vi "Warning Leve Judge.vi"(9 "Limit":T1, 10 "key not found?":bool, 11 "Data":string) -> (2 "level":enum16{"", "Ⅰ", "Ⅱ", "Ⅲ", "Ⅳ", "Ⅴ"}(ring), 3 "字符串":string)   [LabVIEW 2020]
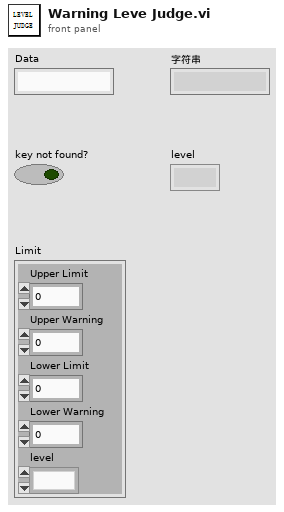
[diagram p1: front panel]
types:
  T1 = cluster{"Upper Limit":dbl, "Upper Warning":dbl, "Lower Limit":dbl, "Lower Warning":dbl, "level":enum16{"", "Ⅰ", "Ⅱ", "Ⅲ", "Ⅳ", "Ⅴ"}}
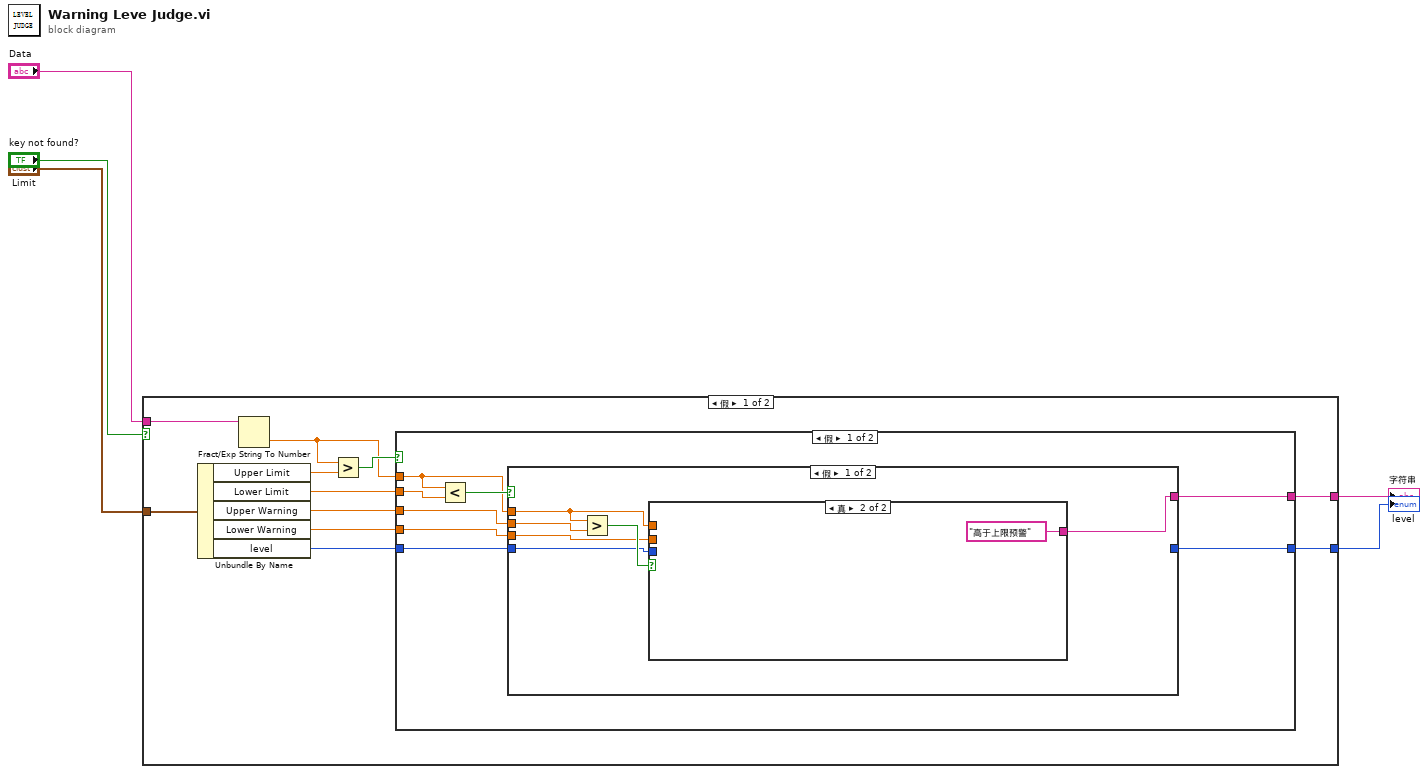
[diagram p0: block diagram]
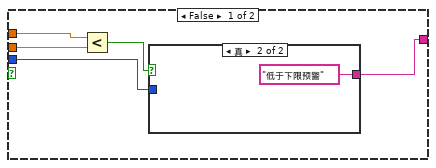
[diagram p2: hidden frame]
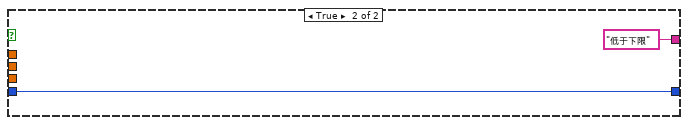
[diagram p4: hidden frame]
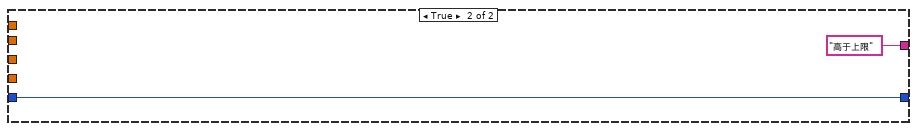
[diagram p5: hidden frame]
diagram:
  n1 = case shown="假" "key not found?" {
    tunnel: "Limit" -> [w16 _]
    tunnel: "Data" -> [w15 _]
    tunnel: [w12 _] -> w3
    tunnel: [w6 _] -> w4
    frame False {
      n2 = Unbundle By Name(w16) -> ("Upper Limit"=w14:dbl, "Lower Limit"=w10:dbl, "Upper Warning"=w9:dbl, "Lower Warning"=w8:dbl, "level"=w7:enum16{"", "Ⅰ", "Ⅱ", "Ⅲ", "Ⅳ", "Ⅴ"})
      n3 = Fract/Exp String To Number(string=w15) -> (number=w11:dbl)  [unwired: 3 in, 1 out]
      n4 = Greater?(x=w11, y=w14) -> (0:w13:bool)
      n5 = case shown="假" w13 {
        tunnel: [w22 "高于上限"] -> w12
        tunnel: w11 -> [w19 _]
        tunnel: w10 -> [w24 _]
        tunnel: w9 -> [w21 _]
        tunnel: w8 -> [w20 _]
        tunnel: w7 -> [w18 w40]
        tunnel: [w17 w40] -> w6
        frame False {
          n6 = Less?(x=w19, y=w24) -> (x < y?=w23:bool)
          n7 = case shown="假" w23 {
            tunnel: [w28 "低于下限"] -> w22
            tunnel: w21 -> [w30 _]
            tunnel: w20 -> [w26 _]
            tunnel: w19 -> [w27 _]
            tunnel: w18 -> [w25 w38]
            tunnel: [_ w38] -> w17
            frame False {
              n8 = Greater?(x=w27, y=w30) -> (0:w29:bool)
              n9 = case shown="真" w29 {
                tunnel: [w32 "高于上限预警"] -> w28
                tunnel: w27 -> [w35 _]
                tunnel: w26 -> [w34 _]
                tunnel: w25 -> [w31 _]
                frame False {
                  n10 = Less?(x=w35, y=w34) -> (x < y?=w33:bool)
                  n11 = case shown="真" w33 {
                    tunnel: [_ "低于下限预警"] -> w32
                    tunnel: w31 -> [_ _]
                    frame False {
                    }
                    frame True {
                    }
                  }
                }
                frame True {
                }
              }
            }
            frame True {
            }
          }
        }
        frame True {
        }
      }
    }
    frame True {
    }
  }
  "level" <- w4
  "字符串" <- w3
